vi "Initialize.vi"(8 "error in":errorcluster, 11 "VI Refnum":refnum<vi>) -> (0 "error out":errorcluster, 3 "Loop Data":T1={"VI Refnum"=refnum, "Timeout"=-1, "Code Data"=[], "Buffer Data"={"Connection ID"=refnum}, "Timer"=4294967295, "Image"=refnum})   [LabVIEW 2016]
uses:
  Data Def/Loop Data.ctl
  Com/Matrix220/Data Def/Com_Matrix220_Buffer Data.ctl
  <vilib>/vision/Image Controls.llb/IMAQ Image.ctl
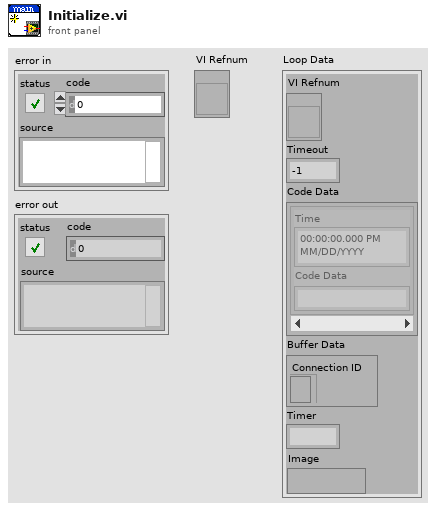
[diagram p1: front panel]
types:
  T1 = typedef "Loop Data.ctl" = cluster{"VI Refnum":refnum<vi>, "Timeout":i32, "Code Data":cluster{"Time":timestamp, "Code Data":string}[], "Buffer Data":T2, "Timer":u32, "Image":T3}
  T2 = typedef "Com_Matrix220_Buffer Data.ctl" = cluster{"Connection ID":refnum<k5>}
  T3 = typedef "IMAQ Image.ctl" = refnum<image>
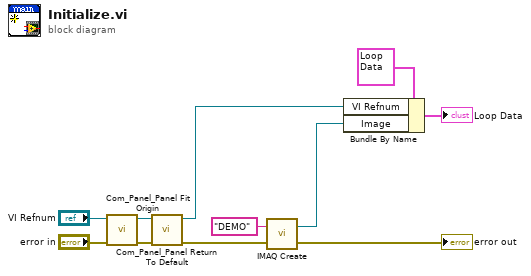
[diagram p0: block diagram]
diagram:
  n1 = call "Com_Panel_Panel Fit Origin.vi"("error in"="error in", "VI Refnum In"="VI Refnum") -> ("error out"=w11:errorcluster, "VI Refnum Out"=w10:refnum<vi>)  [unwired: 8 in]
  n2 = call "Com_Panel_Panel Return To Default.vi"("error in"=w11, "VI Refnum In"=w10) -> ("error out"=w4:errorcluster, "VI Refnum Out"=w6:refnum<vi>)  [unwired: 8 in]
  n3 = call "IMAQ Create"("Image Name"="DEMO", "error in (no error)"=w4) -> ("New Image"=w2:T3, "error out"=→"error out":errorcluster)  [unwired: 3 in]
  n4 = Bundle By Name(cluster=T1 {"VI Refnum"=refnum, "Timeout"=-1, "Code Data"=[], "Buffer Data"={"Connection ID"=refnum}, "Timer"=4294967295, "Image"=refnum} ("Loop Data"), "VI Refnum"=w6, "Image"=w2) -> (→"Loop Data":T1)
